vi "GPS Waypoint List Recorder.vi"(10 "Read Point?":bool, 11 "VISA resource name":refnum<visa-resource-name>) -> ()   [LabVIEW 2009]
uses:
  GPS Read VISA Instance.vi
panel:
  in  "stop":bool
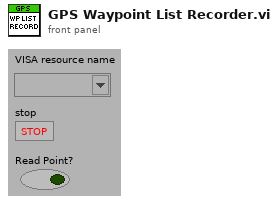
[diagram p1: front panel]
types:
  T1 = enum16{"open", "replace", "create", "open or create", "replace or create", "replace or create with confirmation"}
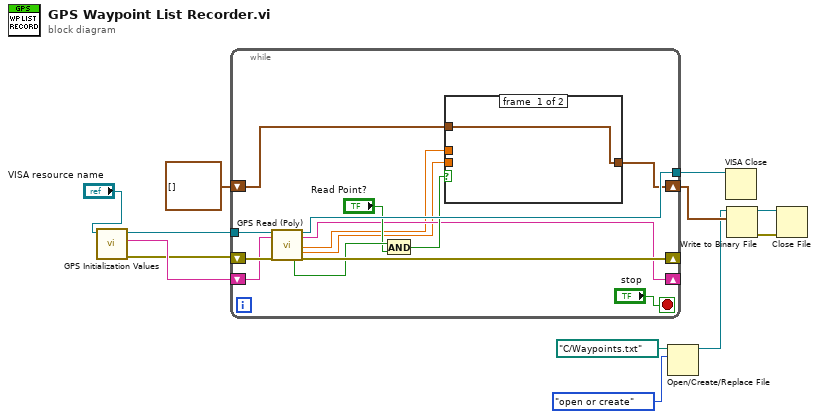
[diagram p0: block diagram]
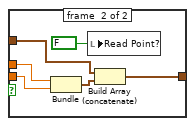
[diagram p2: hidden frame]
diagram:
  n1 = call "GPS Initialization Values.vi"("VISA resource name"="VISA resource name") -> ("error In"=w9:errorcluster, "Buffer In"=w10:string, "VISA resource name In"=w11:refnum<visa-resource-name>)  [unwired: 8 in]
  n2 = while {
    tunnel: [w25] -> w12
    shift-right: [w18] -> _
    shift-left: w10 -> [w19]
    shift-right: [w23] -> _
    shift-left: w9 -> [w24]
    shift-right: [w14] -> w5
    shift-left: cluster{"Longitude":dbl, "Latitude":dbl}[] [] -> [w15]
    tunnel: w11 -> [w13]
    stop <- "stop" stop-if-true
    n3 = call-poly "GPS Read (Poly).vi"("VISA In"=w13, "Buffer In"=w19, "Error In"=w24) -> ("Output Valid?"=w22:bool, "VISA Out"=w25:refnum<visa-resource-name>, "Buffer Out"=w18:string, "Longitude"=w17:dbl, "Latitude"=w16:dbl, "Error Out"=w23:errorcluster)  [unwired: 10 in, 1 out]
    n4 = And(x=w22, y="Read Point?") -> (x .and. y?=w20:bool)
    n5 = case shown="True" w20 {
      tunnel: w17 -> [_ w33]
      tunnel: w16 -> [_ w32]
      tunnel: w15 -> [w27 w31]
      tunnel: [w27 w30] -> w14
      frame #0 {
      }
      frame #1 {
        n6 = Bundle("Longitude"=w33, "Latitude"=w32) -> (w28:cluster{"Longitude":dbl, "Latitude":dbl})  [unwired: 1 in]
        n7 = local write "Read Point?"(FALSE ("Read Point?")) -> ()
        n8 = Build Array (concatenate)(w31, w28) -> (w30:cluster{"Longitude":dbl, "Latitude":dbl}[])
      }
    }
  }
  n9 = Open/Create/Replace File(file path (use dialog)=path "C:/Waypoints.txt", operation (0:open)=T1."open or create") -> (refnum out=w4:refnum<file>)  [unwired: 4 in, 2 out]
  n10 = VISA Close(VISA resource name=w12) -> ()  [unwired: 1 in, 1 out]
  n11 = Write to Binary File(file (use dialog)=w4, data=w5) -> (refnum out=w3:refnum<file>, error out=w2:errorcluster)  [unwired: 4 in, 1 out]
  n12 = Close File(refnum=w3, error in=w2) -> ()  [unwired: 2 out]
